vi "SumpleAudioStart.vi"(3 "microphone settings":T5) -> (1 "All Info":T1 {"Data Set"."Settings"."Time" format="%<%H:%M\n%d/%m/%y>T"; "task ID" format="%.0x"})   [LabVIEW 2014]
uses:
  <userlib>/CurtinCode/AllDataCtrl.ctl
  <userlib>/CurtinCode/DataControl.ctl
  <userlib>/CurtinCode/SettingsControl.ctl
  <vilib>/sound2/lvsound2.llb/Sound Input Task ID.ctl
  <userlib>/CurtinCode/Devicectrl/DeviceData.ctl
  <vilib>/sound2/lvsound2.llb/Sampling Mode.ctl
  <vilib>/sound2/lvsound2.llb/Sound Data Format.ctl
  <userlib>/CurtinCode/Devicectrl/Audio Channel.xctl
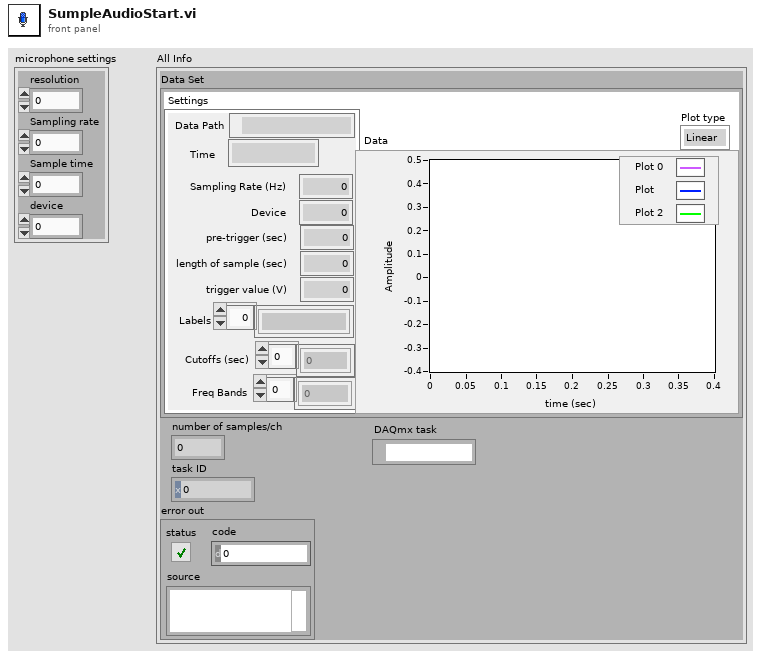
[diagram p1: front panel]
types:
  T1 = typedef "AllDataCtrl.ctl" = cluster{"Data Set":T2, "number of samples/ch":i32, "task ID":T4, "error out":errorcluster, "DAQmx task":refnum<k21>}
  T2 = typedef "DataControl.ctl" = cluster{"Settings":T3, "Data":cluster{i32, dbl, "data":dbl[]}[], "Plot type":enum16{"Linear", "log"}}
  T3 = typedef "SettingsControl.ctl" = cluster{"Data Path":path, "Time":timestamp, "Sampling Rate (Hz)":u16, "Device":u16, "pre-trigger (sec)":dbl, "length of sample (sec)":dbl, "trigger value (V)":dbl, "Labels":string[], "Cutoffs (sec)":dbl[], "Freq Bands":dbl[]}
  T4 = typedef "Sound Input Task ID.ctl" = u32
  T5 = cluster{"resolution":u16, "Sampling rate":u16, "Sample time":dbl, "device":u16}
  T6 = typedef "Audio Channel.xctl/DeviceData.ctl" = cluster{"device ID":u32, "Device Name":string, "number of samples/ch":i32, "sample mode":T7, "sound format":T8, "Sample length (sec)":dbl, "Pre-trigger (sec)":dbl}
  T7 = typedef "Sampling Mode.ctl" = i32
  T8 = typedef "Sound Data Format.ctl" = cluster{"sample rate (S/s)":dbl, "number of channels":i32, "bits per sample":i32}
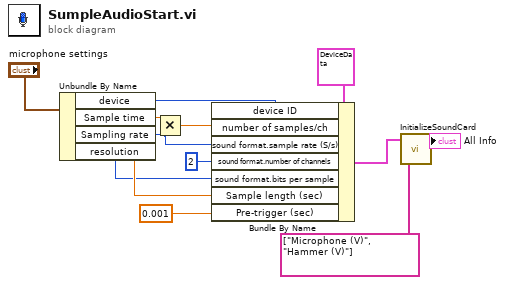
[diagram p0: block diagram]
diagram:
  n1 = Unbundle By Name("microphone settings") -> ("device"=w12:u16, "Sample time"=w6:dbl, "Sampling rate"=w3:u16, "resolution"=w5:u16)
  n2 = Multiply(x=w6, y=w3) -> (x*y=w2:dbl)
  n3 = Bundle By Name(cluster=T6 {"device ID"=0, "Device Name"="", "number of samples/ch"=0, "sample mode"=1, "sound format"={"sample rate (S/s)"=22050.0, "number of channels"=2, "bits per sample"=16}, "Sample length (sec)"=0.5, "Pre-trigger (sec)"=0.1} ("DeviceXControl"), "device ID"=w12, "number of samples/ch"=w2, "sound format.sample rate (S/s)"=w3, "sound format.number of channels"=2, "sound format.bits per sample"=w5, "Sample length (sec)"=w6, "Pre-trigger (sec)"=0.001) -> (w8:T6)
  n4 = call <userlib>:"InitializeSoundCard.vi"("Settings.Labels"=string[] ["Microphone (V)", "Hammer (V)"], "DeviceXControl"=w8) -> ("All Info"=→"All Info":T1)  [unwired: 1 in]
